vi "Default Registry Configuration.vi"() -> (2 "Registry Configuration":T1)   [LabVIEW 2013, in "UniqueName.lvlib" / "NameRegistry.lvclass"]
uses:
  NameRegistry.lvclass
  RegistryConfiguration.ctl
  Delimiter/Delimiter.lvclass
  RandomStringGenerator/RandomStringGenerator.lvclass
  UniquenessCriteria/UniquenessCriteria.lvclass
  StringIncrement/StringIncrement.lvclass
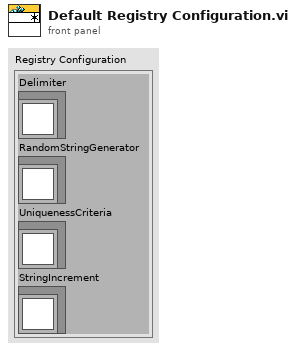
[diagram p1: front panel]
types:
  T1 = typedef "UniqueName.lvlib/NameRegistry.lvclass/RegistryConfiguration.ctl" = cluster{"Delimiter":refnum<class "Delimiter.lvclass">, "RandomStringGenerator":refnum<class "RandomStringGenerator.lvclass">, "UniquenessCriteria":refnum<class "UniquenessCriteria.lvclass">, "StringIncrement":refnum<class "StringIncrement.lvclass">}
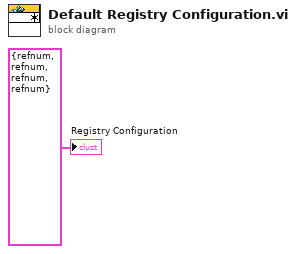
[diagram p0: block diagram]
diagram:
  "Registry Configuration" <- T1 {"Delimiter"=refnum, "RandomStringGenerator"=refnum, "UniquenessCriteria"=refnum, "StringIncrement"=refnum} ("Registry Configuration")
